vi "UpdateOneError.vi"(4 "Description":string, 6 "Library":string, 8 "ErrorIn":errorcluster caption="Error In(no Error)", 9 "Text":string, 10 "ErrorCode":i32, 11 "ReferenceIn":refnum<class "ErrorDefinitionSQLite.lvclass"> caption="Reference In") -> (0 "ErrorOut":errorcluster caption="Error Out", 3 "ReferenceOut":refnum<class "ErrorDefinitionSQLite.lvclass"> caption="Reference Out")   [LabVIEW 2021, in "ErrorDefinitionSQLite.lvclass"]
uses:
  ErrorDefinitionSQLite.lvclass
  <vilib>/drjdpowell/SQLite Library/SQL Connection/Execute SQL.vi
  <vilib>/drjdpowell/SQLite Library/SQLite.lvlib
  <vilib>/drjdpowell/SQLite Library/SQL Connection/Connection.lvclass
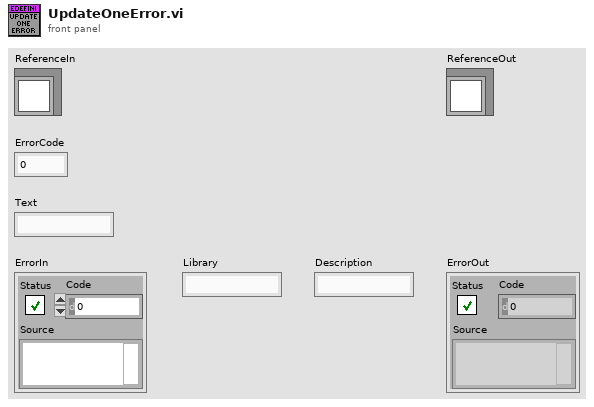
[diagram p1: front panel]
types:
  T1 = typedef "ErrorDefinitionSQLite.lvclass/ObjectAttributes.ctl" = cluster{"Path":path, "SQLiteRef":refnum<class "Connection.lvclass">, "EndOfRange":i32, "DefaultLibrarySize":i32, "StartOfRange":i32}
  T2 = cluster{"Text":string, "Library":string, "Description":string, "App.UserName":string}
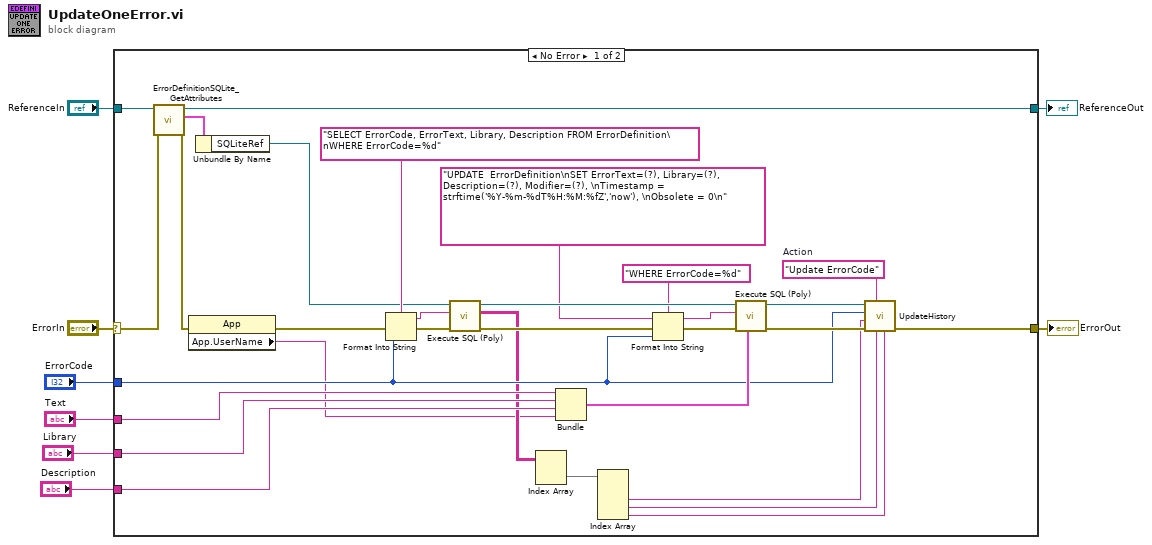
[diagram p0: block diagram]
diagram:
  n1 = case shown="No Error" "ErrorIn" {
    selector: "ErrorIn" -> [w39 w41]
    tunnel: [w9 w41] -> w7
    tunnel: [w37 w40] -> w5
    tunnel: "ReferenceIn" -> [w38 w40]
    tunnel: "ErrorCode" -> [w22 _]
    tunnel: "Text" -> [w29 _]
    tunnel: "Library" -> [w28 _]
    tunnel: "Description" -> [w27 _]
    frame No Error {
      w32 = "Update ErrorCode"  # Action
      n2 = call "ErrorDefinitionSQLite_GetAttributes.vi"("ErrorIn"=w39, "Reference in"=w38) -> ("ErrorOut"=w15:errorcluster, "Data"=w36:T1, "Reference out"=w37:refnum<class "ErrorDefinitionSQLite.lvclass">)  [unwired: 6 in, 1 out]
      n3 = property class="App"(error in=w15) -> (error out=w10:errorcluster, "App.UserName"=w12:string)  [unwired: 1 in, 1 out]
      n4 = Unbundle By Name(w36) -> ("SQLiteRef"=w11:refnum<class "Connection.lvclass">)
      n5 = Format Into String(format string="SELECT ErrorCode, ErrorText, Library, Description FROM ErrorDefinition\nWHERE ErrorCode=%d" ("SQL"), error in=w10, w22) -> (resulting string=w21:string, error out=w23:errorcluster)  [unwired: 1 in]
      n6 = call-poly <vilib>:"Execute SQL (Poly).vi"("error in (no error)"=w23, "SQL"=w21, "SQLite Connection in"=w11) -> ("error out"=w26:errorcluster, "Result Set"=w20:string[][], "SQLite Connection"=w25:refnum<class "Connection.lvclass">)  [unwired: 5 in, 1 out]
      n7 = Index Array(array=w20) -> (element=w19:string[])  [unwired: 2 in]
      n8 = Bundle("Text"=w29, "Library"=w28, "Description"=w27, "App.UserName"=w12) -> (w33:T2)  [unwired: 1 in]
      n9 = Index Array(array=w19) -> (element #2=w18:string, element #3=w17:string, element #4=w16:string)  [unwired: 4 in, 1 out]
      n10 = Format Into String(format string="WHERE ErrorCode=%d" ("SQL"), initial string="UPDATE  ErrorDefinition\nSET ErrorText=(?), Library=(?), Description=(?), Modifier=(?), \nTimestamp = strftime('%Y-%m-%dT%H:%M:%fZ','now'), \nObsolete = 0\n" ("SQL"), error in=w26, w22) -> (resulting string=w34:string, error out=w35:errorcluster)
      n11 = call-poly <vilib>:"Execute SQL (Poly).vi"("Parameter(s)"=w33, "error in (no error)"=w35, "SQL"=w34, "SQLite Connection in"=w25) -> ("error out"=w30:errorcluster, "SQLite Connection"=w31:refnum<class "Connection.lvclass">)  [unwired: 4 in, 2 out]
      n12 = call "UpdateHistory.vi"("Description"=w16, "Library"=w17, "Action"=w32, "error in (no error)"=w30, "ErrorText"=w18, "ErrorCode"=w22, "Connection in"=w31) -> ("error out"=w9:errorcluster)  [unwired: 3 in, 1 out]
    }
    frame Error {
    }
  }
  "ErrorOut" <- w7
  "ReferenceOut" <- w5
